vi "CreateNewWizard_Invoke.vi"(10 "Cluster":T1, 11 "Wizard":T2) -> (3 "Canceled":bool)   [LabVIEW 2020, in "Add Actor.lvlib"]
uses:
  Add Actor.lvlib
  Support/What To Make.ctl
  <resource>/Framework/Providers/API/mxLvNIIM.ctl
  <resource>/Framework/Providers/API/ItemRef.ctl
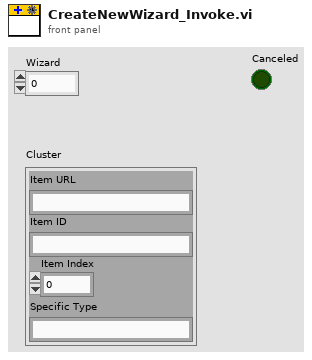
[diagram p1: front panel]
types:
  T1 = typedef "mxLvNIIM.ctl" = cluster{"Item URL":string, "Item ID":string, "Item Index":i32, "Specific Type":string}
  T2 = typedef "ItemRef.ctl" = u64
  T3 = typedef "Add Actor.lvlib/What To Make.ctl" = enum16{"Make Class", "Make Interface"}
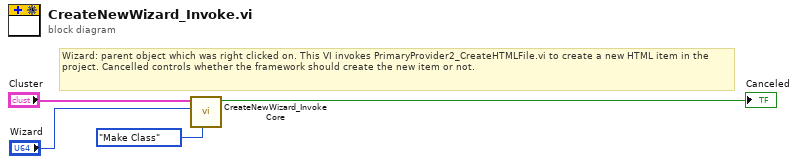
[diagram p0: block diagram]
diagram:
  # "Wizard: parent object which was right clicked on. This VI invokes PrimaryProvider2_CreateHTMLFile.vi to create a new HTML item in the project. Cancelled controls whether the framework should create the new item or not."
  n1 = call "CreateNewWizard_Invoke Core.vi"("what to make"=What_To_Make."Make Class", "Wizard"="Wizard", "Cluster"="Cluster") -> ("Canceled"=→"Canceled":bool)  [unwired: 8 in]
